vi "toBoolean.vi"(11 "String":string) -> (3 "Boolean":bool)   [LabVIEW 2018]
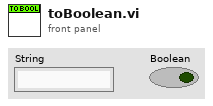
[diagram p1: front panel]
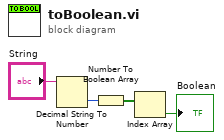
[diagram p0: block diagram]
diagram:
  n1 = Decimal String To Number(string="String") -> (number=w2:i32)  [unwired: 2 in, 1 out]
  n2 = Number To Boolean Array(number=w2) -> (Boolean array=w3:bool[])
  n3 = Index Array(array=w3) -> (element=→"Boolean":bool)  [unwired: 1 in]
